vi "Update Map.vi"(3 "# safety grids":i32=4, 4 "Point":cluster{"Col":i8, "Row":i8}, 5 "Map":i8[][](array[numeric])) -> (1 "Updated Map":i8[][](array[numeric]))   [LabVIEW 2009]
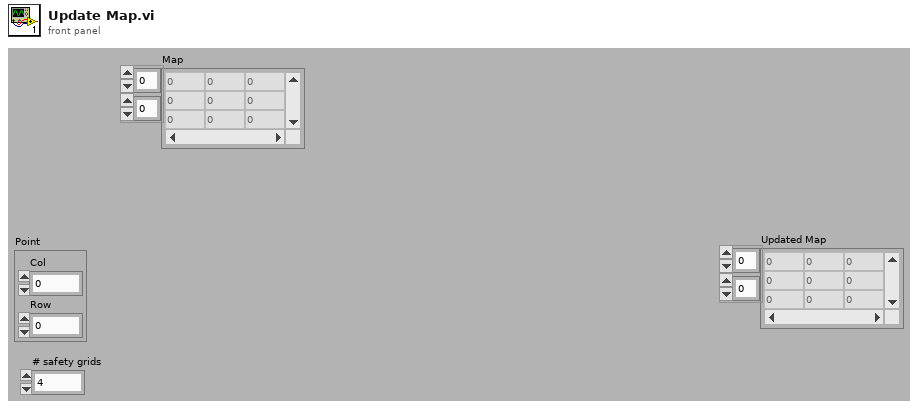
[diagram p1: front panel]
types:
  T1 = typedef "NI_Matrix.lvlib/RealMatrix.ctl" = dbl[][]
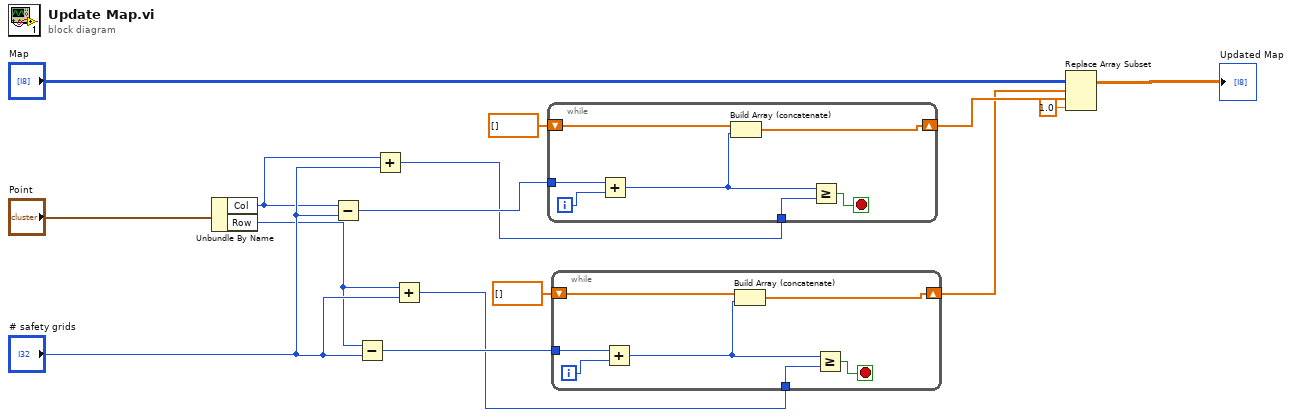
[diagram p0: block diagram]
diagram:
  n1 = Unbundle By Name("Point") -> ("Col"=w12:i8, "Row"=w11:i8)
  n2 = Subtract(x=w12, y="# safety grids") -> (x-y=w8:i32)
  n3 = Subtract(x=w11, y="# safety grids") -> (x-y=w10:i32)
  n4 = Add(x=w12, y="# safety grids") -> (x+y=w7:i32)
  n5 = Add(x=w11, y="# safety grids") -> (x+y=w9:i32)
  n6 = while {
    tunnel: w8 -> [w21]
    tunnel: w7 -> [w17]
    shift-right: [w19] -> w6
    shift-left: dbl[] [] -> [w18]
    i -> [w22]
    stop <- w20 stop-if-true
    n7 = Add(x=w21, y=w22) -> (x+y=w16:i32)
    n8 = Build Array (concatenate)(w18, w16) -> (w19:dbl[])
    n9 = Greater Or Equal?(x=w16, y=w17) -> (x >= y?=w20:bool)
  }
  n10 = while {
    tunnel: w10 -> [w28]
    tunnel: w9 -> [w24]
    shift-right: [w26] -> w5
    shift-left: dbl[] [] -> [w25]
    i -> [w29]
    stop <- w27 stop-if-true
    n11 = Add(x=w28, y=w29) -> (x+y=w23:i32)
    n12 = Build Array (concatenate)(w25, w23) -> (w26:dbl[])
    n13 = Greater Or Equal?(x=w23, y=w24) -> (x >= y?=w27:bool)
  }
  n14 = Replace Array Subset(array="Map", new element=1.0 ("new element/submatrix"), index (row)=w5, index (col)=w6) -> (→"Updated Map":T1)
